vi "LVClass_ClosedLoopSecurityActivation_Ctor_FromHighDefaultParams.vi"(0 "ClosedLoopSecurity (const)":refnum<class "ClosedLoopSecurityActivation.lvclass">, 11 "error in (no error)":errorcluster) -> (4 "ClosedLoopSecurity (new)":refnum<class "ClosedLoopSecurityActivation.lvclass">, 15 "error out":errorcluster)   [LabVIEW 2020, in "ClosedLoopSecurityActivation.lvclass"]
doc: "Construction from Imagine Optic recommended high security activations.\n\n<B>security_activationIn</B> : Constant Pointer to Closed Loop security activation object.\n<B>security_activationOut</B> : Constant Pointer to Closed Loop security activation object."
uses:
  ClosedLoopSecurityActivation.lvclass
  Controls/Handle creation.ctl
  ClosedLoopSecurityActivation.lvclass/ClosedLoopSecurityActivation.ctl
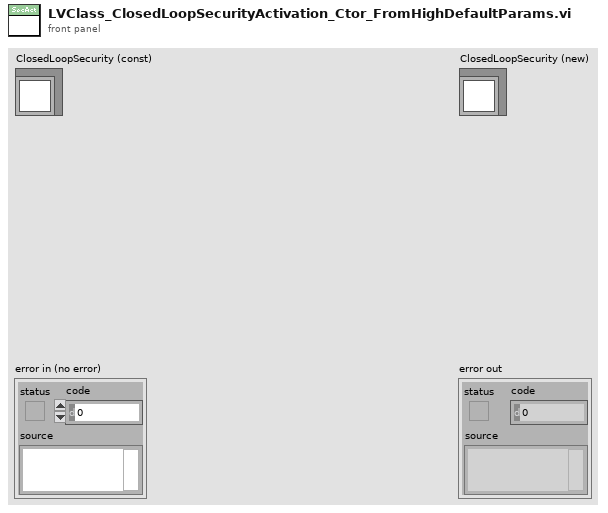
[diagram p1: front panel]
types:
  T1 = typedef "Handle creation.ctl" = enum16{"By ctor", "By write function"}
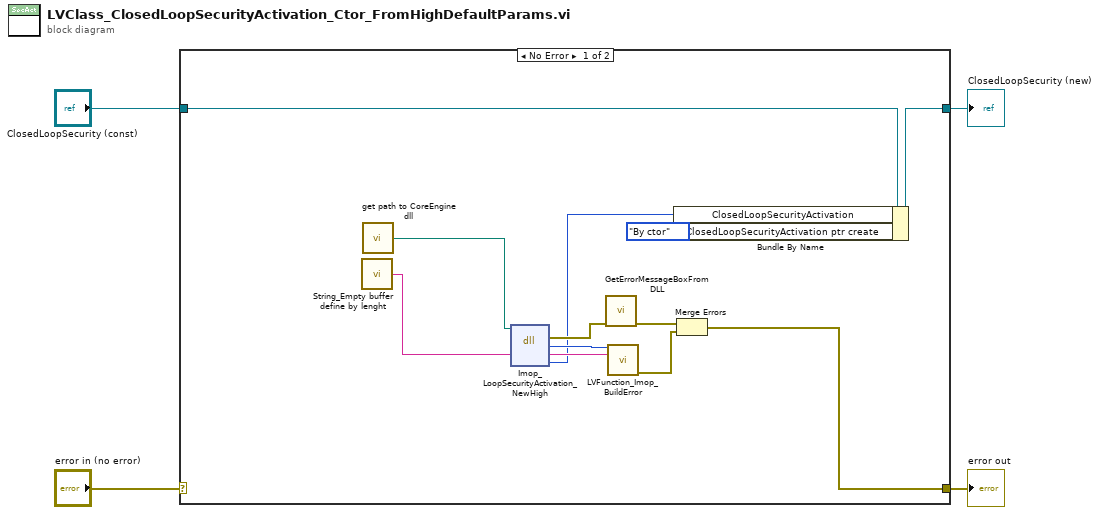
[diagram p0: block diagram]
diagram:
  n1 = case shown="No Error" "error in (no error)" {
    selector: "error in (no error)" -> [_ w18]
    tunnel: [w5 w18] -> w3
    tunnel: [w6 w17] -> w1
    tunnel: "ClosedLoopSecurity (const)" -> [w7 w17]
    frame No Error {
      n2 = call "String_Empty buffer define by lenght.vi"() -> ("Empty buffer"=w16:string)  [unwired: 1 in]
      n3 = call "get path to CoreEngine dll.vi"() -> ("path to wavekit library"=w8:path)  [unwired: 14 in, 1 out]
      n4 = dll-call lib="D:/soft/HASO_v3/SVN_trunk/ImOpCoreEngine4_LV2011/DLLs/c_interface_vc100.dll" fn="Imop_LoopSecurityActivation_NewHigh"(path in=w8, "message"=w16) -> (error out=w13:errorcluster, "return type"=w14:i32, "message"=w15:string, "security_activation"=w12:i64)  [unwired: 3 in, 1 out]
      n5 = call "GetErrorMessageBoxFromDLL.vi"("error IN"=w13) -> ("error OUT"=w10:errorcluster)  [unwired: 10 in]
      n6 = call "LVFunction_Imop_BuildError.vi"("code"=w14, "String to Prepend to source (\"\")"=w15) -> ("error out"=w9:errorcluster)  [unwired: 13 in]
      n7 = Bundle By Name(cluster=w7, "ClosedLoopSecurityActivation"=w12, "ClosedLoopSecurityActivation ptr create"=Handle_creation."By ctor" ("Pupil ptr create")) -> (w6:refnum<class "ClosedLoopSecurityActivation.lvclass">)
      n8 = Merge Errors(w10, w9) -> (w5:errorcluster)
    }
    frame Error {
    }
  }
  "error out" <- w3
  "ClosedLoopSecurity (new)" <- w1
